vi "Test_Multiple_SubPanel_Self_Control.vi"() -> ()   [LabVIEW 2021]
panel:
  out "Total_State":i32 caption="Total Independent State Object"
  in  "Show Stop Button":bool
  in  "UnLoad_Panel":bool
  in  "Load_Panel":bool
  in  "Time Target (s)":dbl=30.0 format="%#_13g"
  in  "System_Delay(s)":dbl=0.01 format="%.0p"
  in  "State_Interval_Time(s)":dbl format="%.0p"
  in  "State#":i32=100
  in  "Stop":bool
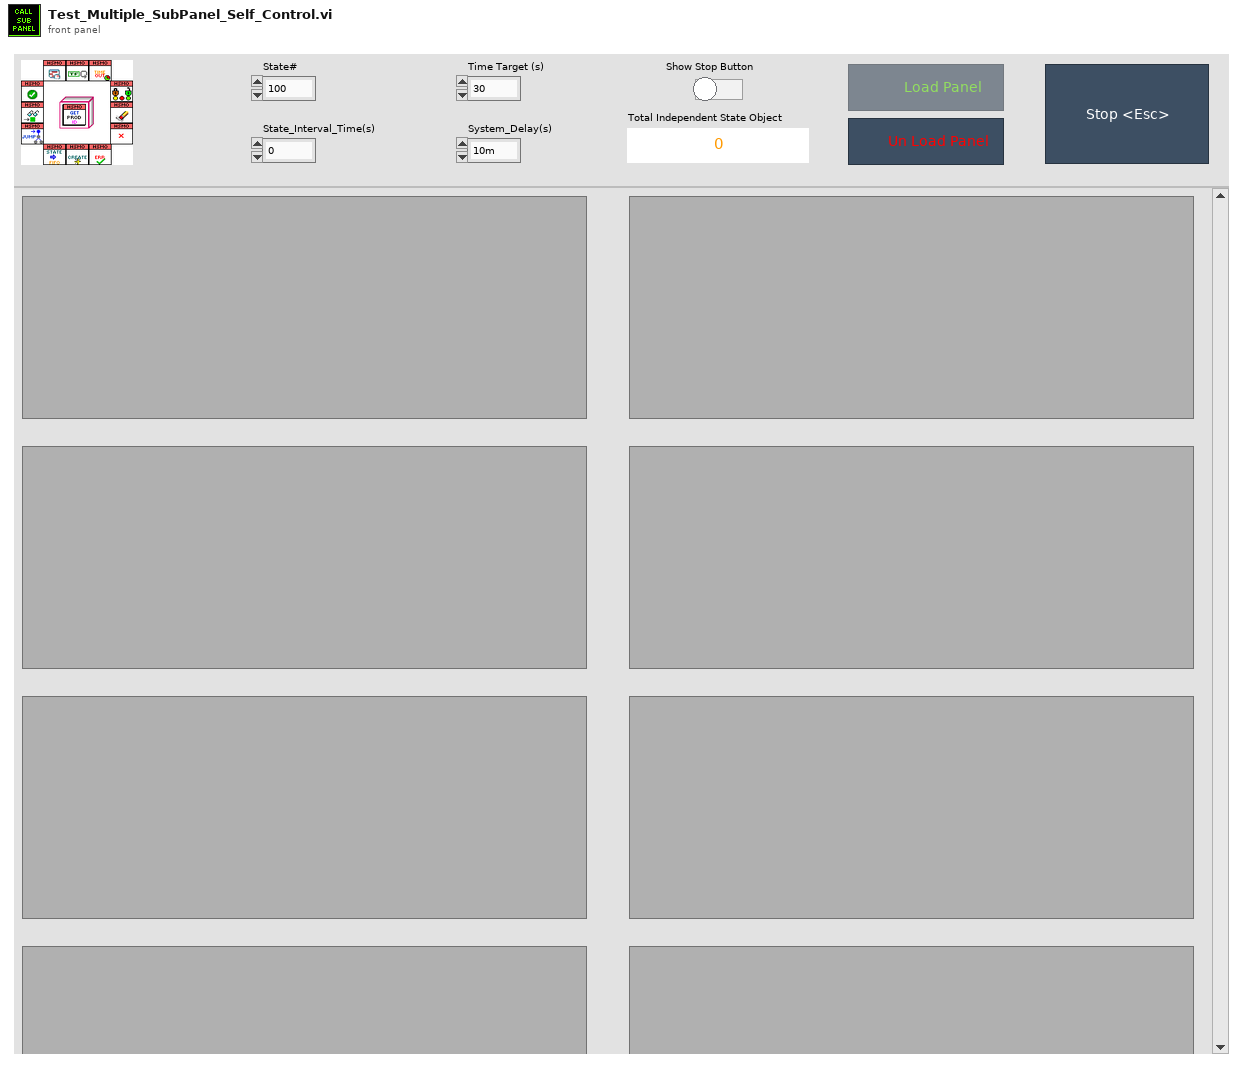
[diagram p1: front panel]
types:
  T1 = enum8{"Enabled", "Disabled", "Disabled and Grayed Out"}
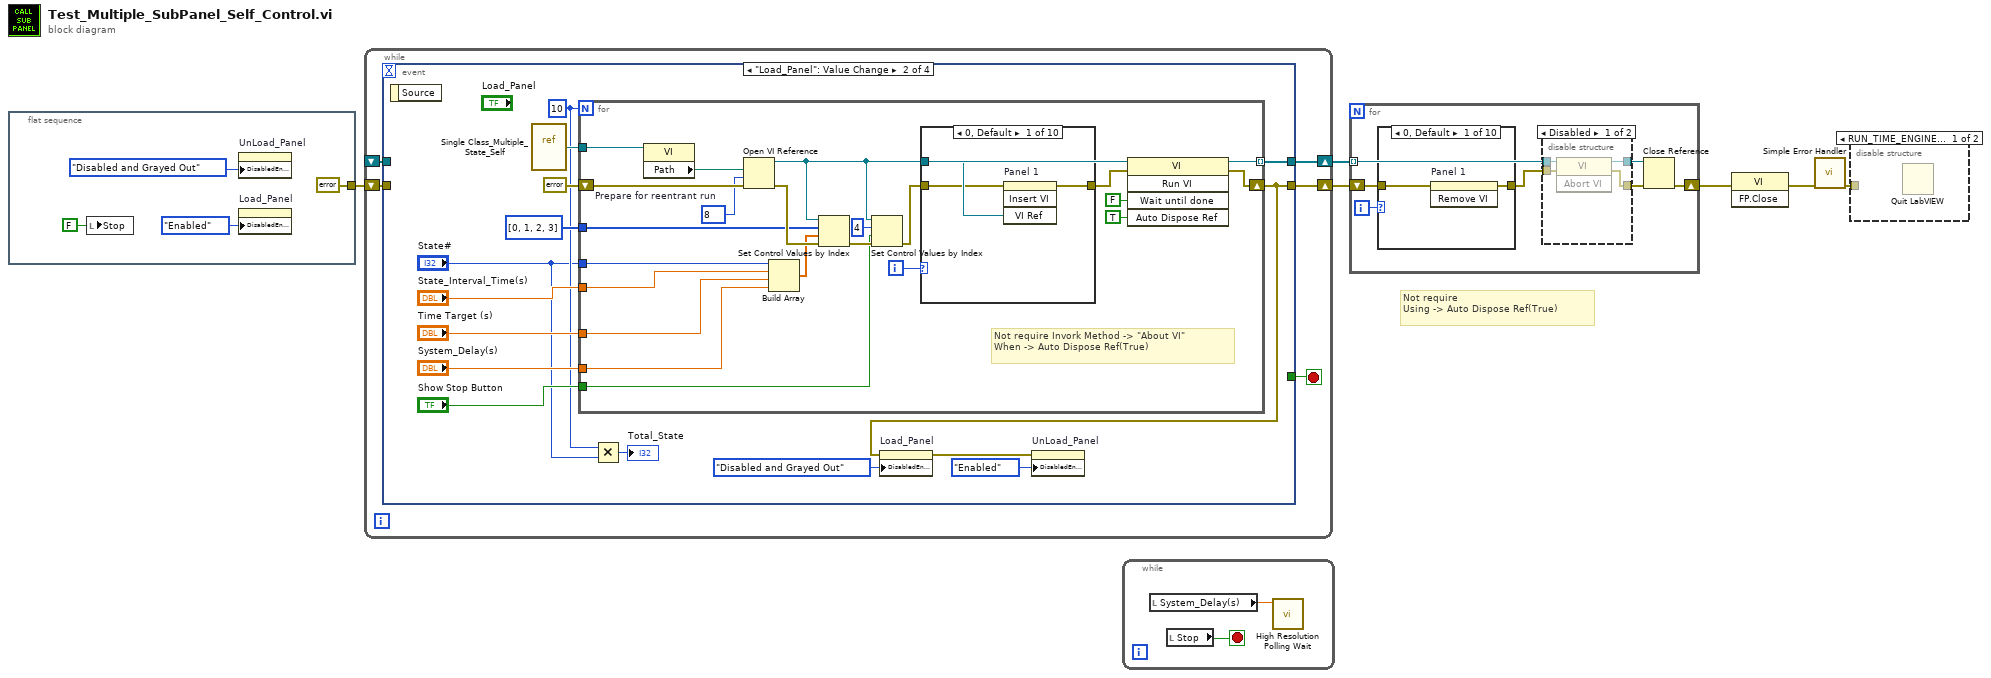
[diagram p0: block diagram]
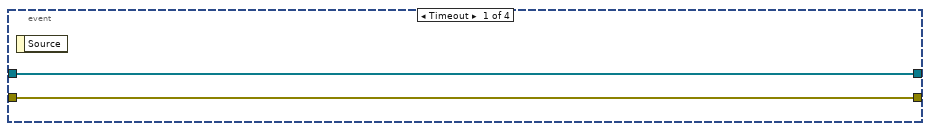
[diagram p3: hidden frame]
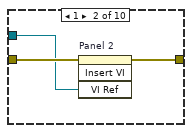
[diagram p4: hidden frame]
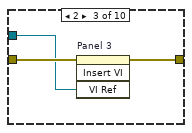
[diagram p5: hidden frame]
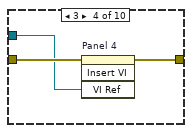
[diagram p6: hidden frame]
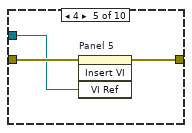
[diagram p7: hidden frame]
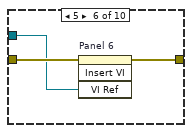
[diagram p8: hidden frame]
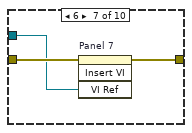
[diagram p9: hidden frame]
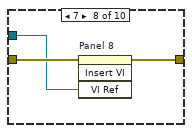
[diagram p10: hidden frame]
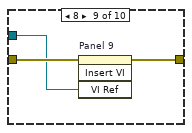
[diagram p11: hidden frame]
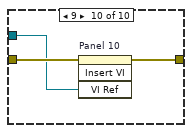
[diagram p12: hidden frame]
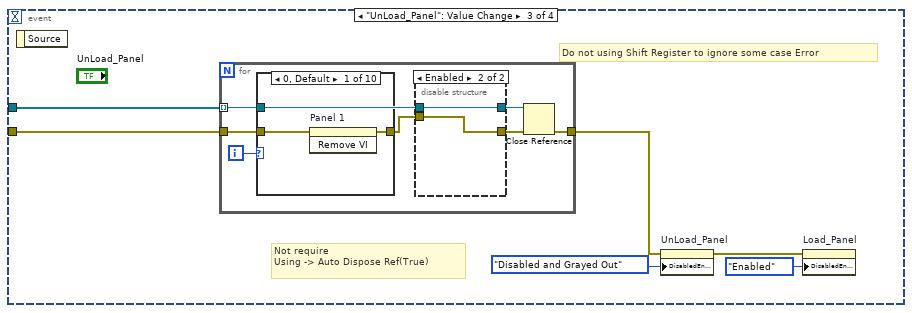
[diagram p13: hidden frame]
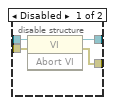
[diagram p14: hidden frame]
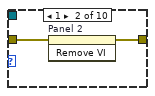
[diagram p15: hidden frame]
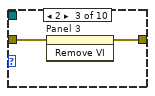
[diagram p16: hidden frame]
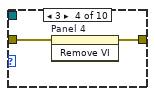
[diagram p17: hidden frame]
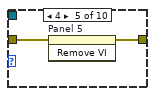
[diagram p18: hidden frame]
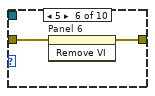
[diagram p19: hidden frame]
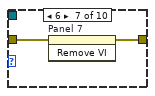
[diagram p20: hidden frame]
diagram:
  # "Not require\nUsing -> Auto Dispose Ref(True)"
  n1 = flat-sequence {
    tunnel: [errorcluster {"status"=FALSE, "code"=0, "source"=""} ("error out")] -> w4
    frame #0 {
      n2 = local write "Stop"(FALSE ("Stop")) -> ()
      n3 = property on="UnLoad_Panel" class="Bool"("DisabledEnum"=T1."Disabled and Grayed Out" ("Disabled")) -> ()  [unwired: 2 in, 2 out]
      n4 = property on="Load_Panel" class="Bool"("DisabledEnum"=T1."Enabled" ("Disabled")) -> ()  [unwired: 2 in, 2 out]
    }
  }
  n5 = while {
    shift-right: [w14] -> w6
    shift-left: _ -> [w13]
    shift-right: [w12] -> w5
    shift-left: w4 -> [w11]
    stop <- w15 stop-if-true
    n6 = event shown="[1] \"Load_Panel\": Value Change" {
      selector: _ -> [_ _ _ _]
      dyn-events: _ -> [_ _ _ _]
      timeout: _ -> [_ _ _ _]
      tunnel: [_ _ _ w125] -> w15
      tunnel: [w17 w26 _ w126] -> w14
      tunnel: w13 -> [w17 _ w90 w126]
      tunnel: [w16 w21 _ w124] -> w12
      tunnel: w11 -> [w16 _ w86 w124]
      event Timeout {
        n7 = event-data() -> ()  [unwired: 1 in, 1 out]
      }
      event "Load_Panel": Value Change {
        w19 = 10
        n8 = event-data() -> ()  [unwired: 1 in, 1 out]
        n9 = vi-ref "Single Class_Multiple_State_Self.vi"() -> (w32:refnum<vi>)
        n10 = for {
          N: w19 -> [_]
          shift-right: [w43] -> w21
          shift-left: errorcluster {"status"=FALSE, "code"=0, "source"=""} ("error out") -> [w53]
          tunnel: w32 -> [w52]
          tunnel: [w45] -> w26 mode=indexing
          tunnel: "State_Interval_Time(s)" -> [w38]
          tunnel: "State#" -> [w37]
          tunnel: "System_Delay(s)" -> [w36]
          tunnel: "Time Target (s)" -> [w35]
          tunnel: i32[] [0, 1, 2, 3] ("control indexes") -> [w34]
          tunnel: "Show Stop Button" -> [w33]
          i -> [w51]
          w50 = 8  # Prepare for reentrant run
          # "Not require Invork Method -> \"About VI\"\nWhen -> Auto Dispose Ref(True)"
          n11 = property class="VI"(reference=w52) -> ("Path"=w54:path)  [unwired: 1 in, 2 out]
          n12 = Open VI Reference(vi path=w54, options=w50, error in (no error)=w53) -> (vi reference=w39:refnum<vi>, error out=w49:errorcluster)  [unwired: 3 in]
          n13 = Build Array(w37, w38, w35, w36) -> (w42:dbl[])
          n14 = Set Control Values by Index(0:w39, 1:w34, 2:w42, 3:w49) -> (11:w41:errorcluster)
          n15 = Set Control Values by Index(0:w39, 1:4, 2:w33, 3:w41) -> (11:w48:errorcluster)
          n16 = case shown="0, Default" w51 {
            tunnel: w48 -> [w55 w60 w63 w66 w69 w72 w75 w78 w81 w84]
            tunnel: w39 -> [w56 w59 w61 w64 w67 w70 w73 w76 w79 w82]
            tunnel: [w57 w58 w62 w65 w68 w71 w74 w77 w80 w83] -> w44
            frame 0, Default {
              n17 = invoke on="Panel 1" class="SubPnl" method="Insert VI"(error in=w55, "VI Ref"=w56) -> (error out=w57:errorcluster)  [unwired: 2 in, 3 out]
            }
            frame 1 {
              n18 = invoke on="Panel 2" class="SubPnl" method="Insert VI"(error in=w60, "VI Ref"=w59) -> (error out=w58:errorcluster)  [unwired: 2 in, 3 out]
            }
            frame 2 {
              n19 = invoke on="Panel 3" class="SubPnl" method="Insert VI"(error in=w63, "VI Ref"=w61) -> (error out=w62:errorcluster)  [unwired: 2 in, 3 out]
            }
            frame 3 {
              n20 = invoke on="Panel 4" class="SubPnl" method="Insert VI"(error in=w66, "VI Ref"=w64) -> (error out=w65:errorcluster)  [unwired: 2 in, 3 out]
            }
            frame 4 {
              n21 = invoke on="Panel 5" class="SubPnl" method="Insert VI"(error in=w69, "VI Ref"=w67) -> (error out=w68:errorcluster)  [unwired: 2 in, 3 out]
            }
            frame 5 {
              n22 = invoke on="Panel 6" class="SubPnl" method="Insert VI"(error in=w72, "VI Ref"=w70) -> (error out=w71:errorcluster)  [unwired: 2 in, 3 out]
            }
            frame 6 {
              n23 = invoke on="Panel 7" class="SubPnl" method="Insert VI"(error in=w75, "VI Ref"=w73) -> (error out=w74:errorcluster)  [unwired: 2 in, 3 out]
            }
            frame 7 {
              n24 = invoke on="Panel 8" class="SubPnl" method="Insert VI"(error in=w78, "VI Ref"=w76) -> (error out=w77:errorcluster)  [unwired: 2 in, 3 out]
            }
            frame 8 {
              n25 = invoke on="Panel 9" class="SubPnl" method="Insert VI"(error in=w81, "VI Ref"=w79) -> (error out=w80:errorcluster)  [unwired: 2 in, 3 out]
            }
            frame 9 {
              n26 = invoke on="Panel 10" class="SubPnl" method="Insert VI"(error in=w84, "VI Ref"=w82) -> (error out=w83:errorcluster)  [unwired: 2 in, 3 out]
            }
          }
          n27 = invoke class="VI" method="Run VI"(reference=w39, error in=w44, "Wait until done"=FALSE ("Wait Until Done"), "Auto Dispose Ref"=TRUE ("Auto Dispose Reference")) -> (reference out=w45:refnum<vi>, error out=w43:errorcluster)  [unwired: 1 in, 3 out]
        }
        n28 = Multiply(x=w19, y="State#") -> (x*y=→"Total_State":i32)
        n29 = property on="Load_Panel" class="Bool"(error in=w21, "DisabledEnum"=T1."Disabled and Grayed Out" ("Disabled")) -> (error out=w22:errorcluster)  [unwired: 1 in, 1 out]
        n30 = property on="UnLoad_Panel" class="Bool"(error in=w22, "DisabledEnum"=T1."Enabled" ("Disabled")) -> ()  [unwired: 1 in, 2 out]
      }
      event "UnLoad_Panel": Value Change {
        # "Do not using Shift Register to ignore some case Error"
        # "Not require\nUsing -> Auto Dispose Ref(True)"
        n31 = event-data() -> ()  [unwired: 1 in, 1 out]
        n32 = for {
          tunnel: w90 -> [w95] mode=indexing
          tunnel: w86 -> [w92]
          tunnel: [w91] -> w85
          i -> [w94]
          n33 = case shown="0, Default" w94 {
            tunnel: w92 -> [w104 w107 w109 w111 w113 w115 w117 w119 w121 w123]
            tunnel: w95 -> [_ _ _ _ _ _ _ _ _ _]
            tunnel: [w105 w106 w108 w110 w112 w114 w116 w118 w120 w122] -> w93
            frame 0, Default {
              n34 = invoke on="Panel 1" class="SubPnl" method="Remove VI"(error in=w104) -> (error out=w105:errorcluster)  [unwired: 2 in, 2 out]
            }
            frame 1 {
              n35 = invoke on="Panel 2" class="SubPnl" method="Remove VI"(error in=w107) -> (error out=w106:errorcluster)  [unwired: 2 in, 2 out]
            }
            frame 2 {
              n36 = invoke on="Panel 3" class="SubPnl" method="Remove VI"(error in=w109) -> (error out=w108:errorcluster)  [unwired: 2 in, 2 out]
            }
            frame 3 {
              n37 = invoke on="Panel 4" class="SubPnl" method="Remove VI"(error in=w111) -> (error out=w110:errorcluster)  [unwired: 2 in, 2 out]
            }
            frame 4 {
              n38 = invoke on="Panel 5" class="SubPnl" method="Remove VI"(error in=w113) -> (error out=w112:errorcluster)  [unwired: 2 in, 2 out]
            }
            frame 5 {
              n39 = invoke on="Panel 6" class="SubPnl" method="Remove VI"(error in=w115) -> (error out=w114:errorcluster)  [unwired: 2 in, 2 out]
            }
            frame 6 {
              n40 = invoke on="Panel 7" class="SubPnl" method="Remove VI"(error in=w117) -> (error out=w116:errorcluster)  [unwired: 2 in, 2 out]
            }
            frame 7 {
              n41 = invoke on="Panel 8" class="SubPnl" method="Remove VI"(error in=w119) -> (error out=w118:errorcluster)  [unwired: 2 in, 2 out]
            }
            frame 8 {
              n42 = invoke on="Panel 9" class="SubPnl" method="Remove VI"(error in=w121) -> (error out=w120:errorcluster)  [unwired: 2 in, 2 out]
            }
            frame 9 {
              n43 = invoke on="Panel 10" class="SubPnl" method="Remove VI"(error in=w123) -> (error out=w122:errorcluster)  [unwired: 2 in, 2 out]
            }
          }
          n44 = disable-structure shown="Enabled" {
            disable-tunnel: [w101 w103] -> w97
            disable-tunnel: [w100 w102] -> w96
            disable-tunnel: w95 -> [w99 w103]
            disable-tunnel: w93 -> [w98 w102]
            frame Disabled {
              n45 = invoke class="VI" method="Abort VI"(reference=w99, error in=w98) -> (reference out=w101:refnum<vi>, error out=w100:errorcluster)  [unwired: 1 in, 1 out]
            }
            frame Enabled {
            }
          }
          n46 = Close Reference(reference=w97, error in (no error)=w96) -> (error out=w91:errorcluster)
        }
        n47 = property on="UnLoad_Panel" class="Bool"(error in=w85, "DisabledEnum"=T1."Disabled and Grayed Out" ("Disabled")) -> (error out=w87:errorcluster)  [unwired: 1 in, 1 out]
        n48 = property on="Load_Panel" class="Bool"(error in=w87, "DisabledEnum"=T1."Enabled" ("Disabled")) -> ()  [unwired: 1 in, 2 out]
      }
      event "Stop": Value Change {
        n49 = event-data() -> ()  [unwired: 1 in, 1 out]
        n50 = Two Button Dialog(message="Exit Confirm !") -> (T button?=w125:bool)  [unwired: 2 in]
        n51 = local write "Stop"(w125) -> ()
      }
    }
  }
  n52 = while {
    stop <- w128 stop-if-true
    n53 = local read "System_Delay(s)"() -> (w129:dbl)
    n54 = local read "Stop"() -> (w128:bool)
    n55 = call <vilib>:"High Resolution Polling Wait.vi"("seconds to wait"=w129) -> ()  [unwired: 10 in, 1 out]
  }
  n56 = for {
    tunnel: w6 -> [w136] mode=indexing
    shift-right: [w133] -> w2
    shift-left: w5 -> [w132]
    i -> [w131]
    n57 = case shown="0, Default" w131 {
      tunnel: w132 -> [w143 w146 w148 w150 w152 w154 w156 w158 w160 w162]
      tunnel: [w144 w145 w147 w149 w151 w153 w155 w157 w159 w161] -> w130
      frame 0, Default {
        n58 = invoke on="Panel 1" class="SubPnl" method="Remove VI"(error in=w143) -> (error out=w144:errorcluster)  [unwired: 2 in, 2 out]
      }
      frame 1 {
        n59 = invoke on="Panel 2" class="SubPnl" method="Remove VI"(error in=w146) -> (error out=w145:errorcluster)  [unwired: 2 in, 2 out]
      }
      frame 2 {
        n60 = invoke on="Panel 3" class="SubPnl" method="Remove VI"(error in=w148) -> (error out=w147:errorcluster)  [unwired: 2 in, 2 out]
      }
      frame 3 {
        n61 = invoke on="Panel 4" class="SubPnl" method="Remove VI"(error in=w150) -> (error out=w149:errorcluster)  [unwired: 2 in, 2 out]
      }
      frame 4 {
        n62 = invoke on="Panel 5" class="SubPnl" method="Remove VI"(error in=w152) -> (error out=w151:errorcluster)  [unwired: 2 in, 2 out]
      }
      frame 5 {
        n63 = invoke on="Panel 6" class="SubPnl" method="Remove VI"(error in=w154) -> (error out=w153:errorcluster)  [unwired: 2 in, 2 out]
      }
      frame 6 {
        n64 = invoke on="Panel 7" class="SubPnl" method="Remove VI"(error in=w156) -> (error out=w155:errorcluster)  [unwired: 2 in, 2 out]
      }
      frame 7 {
        n65 = invoke on="Panel 8" class="SubPnl" method="Remove VI"(error in=w158) -> (error out=w157:errorcluster)  [unwired: 2 in, 2 out]
      }
      frame 8 {
        n66 = invoke on="Panel 9" class="SubPnl" method="Remove VI"(error in=w160) -> (error out=w159:errorcluster)  [unwired: 2 in, 2 out]
      }
      frame 9 {
        n67 = invoke on="Panel 10" class="SubPnl" method="Remove VI"(error in=w162) -> (error out=w161:errorcluster)  [unwired: 2 in, 2 out]
      }
    }
    n68 = disable-structure shown="Disabled" {
      disable-tunnel: w136 -> [w140 w142]
      disable-tunnel: [w139 w142] -> w135
      disable-tunnel: [w138 w141] -> w134
      disable-tunnel: w130 -> [w137 w141]
      frame Disabled {
        n69 = invoke class="VI" method="Abort VI"(reference=w140, error in=w137) -> (reference out=w139:refnum<vi>, error out=w138:errorcluster)  [unwired: 1 in, 1 out]
      }
      frame Enabled {
      }
    }
    n70 = Close Reference(reference=w135, error in (no error)=w134) -> (error out=w133:errorcluster)
  }
  n71 = invoke class="VI" method="FP.Close"(error in=w2) -> (error out=w3:errorcluster)  [unwired: 2 in, 2 out]
  n72 = call <vilib>:"Simple Error Handler.vi"("error in (no error)"=w3) -> ("error out"=w1:errorcluster)  [unwired: 4 in, 4 out]
  n73 = disable-structure shown="RUN_TIME_ENGINE==True" {
    disable-tunnel: w1 -> [_ _]
    frame condition #0 {
      n74 = Quit LabVIEW() -> ()  [unwired: 1 in]
    }
    frame condition #1 (active) {
    }
  }
